vi "Build Rx UDP Engine Configuration.vi"(0 "section ref in":T8=18446744073709551615 format="%.0x", 5 "board properties":T6 {"portConfig" items=["FDX_SINGLE", "FDX_REDUNDANT"]; "portSpeed" items=["FDX_100MBIT", "FDX_10MBIT", "FDX_AUTO_100MBIT", "FDX_AUTO_10MBIT", "FDX_AUTO_ERROR", "FDX_1000MBIT"]}, 9 "port properties":T5, 11 "error in":errorcluster) -> (4 "section ref out":T8 format="%.0x", 6 "boardId":u32, 8 "portId":u32, 10 "VL Configurations":T7(array[cluster]) {"VL Config"."FilterMode" items=["FDX_RX_VL_FLT_DIS", "FDX_RX_VL_FLT_ENA ", "FDX_RX_VL_FLT_ENA_INV"]; "VL Config"."VLBufSize" format="%.0x"; "VL Config"."VerificationMode" items=["FDX_RX_VL_CHECK_ENA_DEFAULT"=65535, "FDX_RX_VL_CHECK_REDMAM"=16, "DX_RX_VL_CHECK_TRAFIC"=8, "FDX_RX_VL_CHECK_FRAMESIZE"=4, "FDX_RX_VL_CHECK_SNINTEG"=2, "FDX_RX_VL_CHECK_INVPAC"=1, "FDX_RX_VL_CHECK_DISA"=0]}, 14 "CommPort Payload":T3[](array[typedef]) {"Parameters"."encoding" items=["BNR", "BCD", "Discrete", "Signed_32", "Signed_64", "Float_32", "Float_64", "Opaque"]}, 15 "error out":errorcluster)   [LabVIEW 2020, in "AIM ARINC 664 Scripting.lvlib"]
uses:
  AIM ARINC 664 Scripting.lvlib
  <vilib>/NI VeriStand/Custom Device API/Custom Device API.lvlib
  Program Files/National Instruments/LabVIEW 2025/instr.lib/AIM GmbH/_AIM 664/_controls/comm_udp_rx.ctl
  Program Files/National Instruments/LabVIEW 2025/instr.lib/AIM GmbH/_AIM 664/AIM664LV.lvlib
  Program Files/National Instruments/LabVIEW 2025/instr.lib/AIM GmbH/_AIM 664/_controls/comm_verification_rx.ctl
  Shared/Encoding (Arinc664).ctl
  Import/_typedefs/frame_parameter_definition.ctl
  Import/AIM ARINC 664 Import.lvlib
  Shared/rx_udp_payload_config.ctl
  <vilib>/NI VeriStand/Custom Device API/Custom Device Item Ref.ctl
  Import/_typedefs/board_setup.ctl
  Import/_typedefs/port_setup.ctl
panel:
  in  "Cluster":cluster{"VL Config":T1, "CommPort Config":T2[]} {"VL Config"."FilterMode" items=["FDX_RX_VL_FLT_DIS", "FDX_RX_VL_FLT_ENA ", "FDX_RX_VL_FLT_ENA_INV"]; "VL Config"."VLBufSize" format="%.0x"; "VL Config"."VerificationMode" items=["FDX_RX_VL_CHECK_ENA_DEFAULT"=65535, "FDX_RX_VL_CHECK_REDMAM"=16, "DX_RX_VL_CHECK_TRAFIC"=8, "FDX_RX_VL_CHECK_FRAMESIZE"=4, "FDX_RX_VL_CHECK_SNINTEG"=2, "FDX_RX_VL_CHECK_INVPAC"=1, "FDX_RX_VL_CHECK_DISA"=0]}
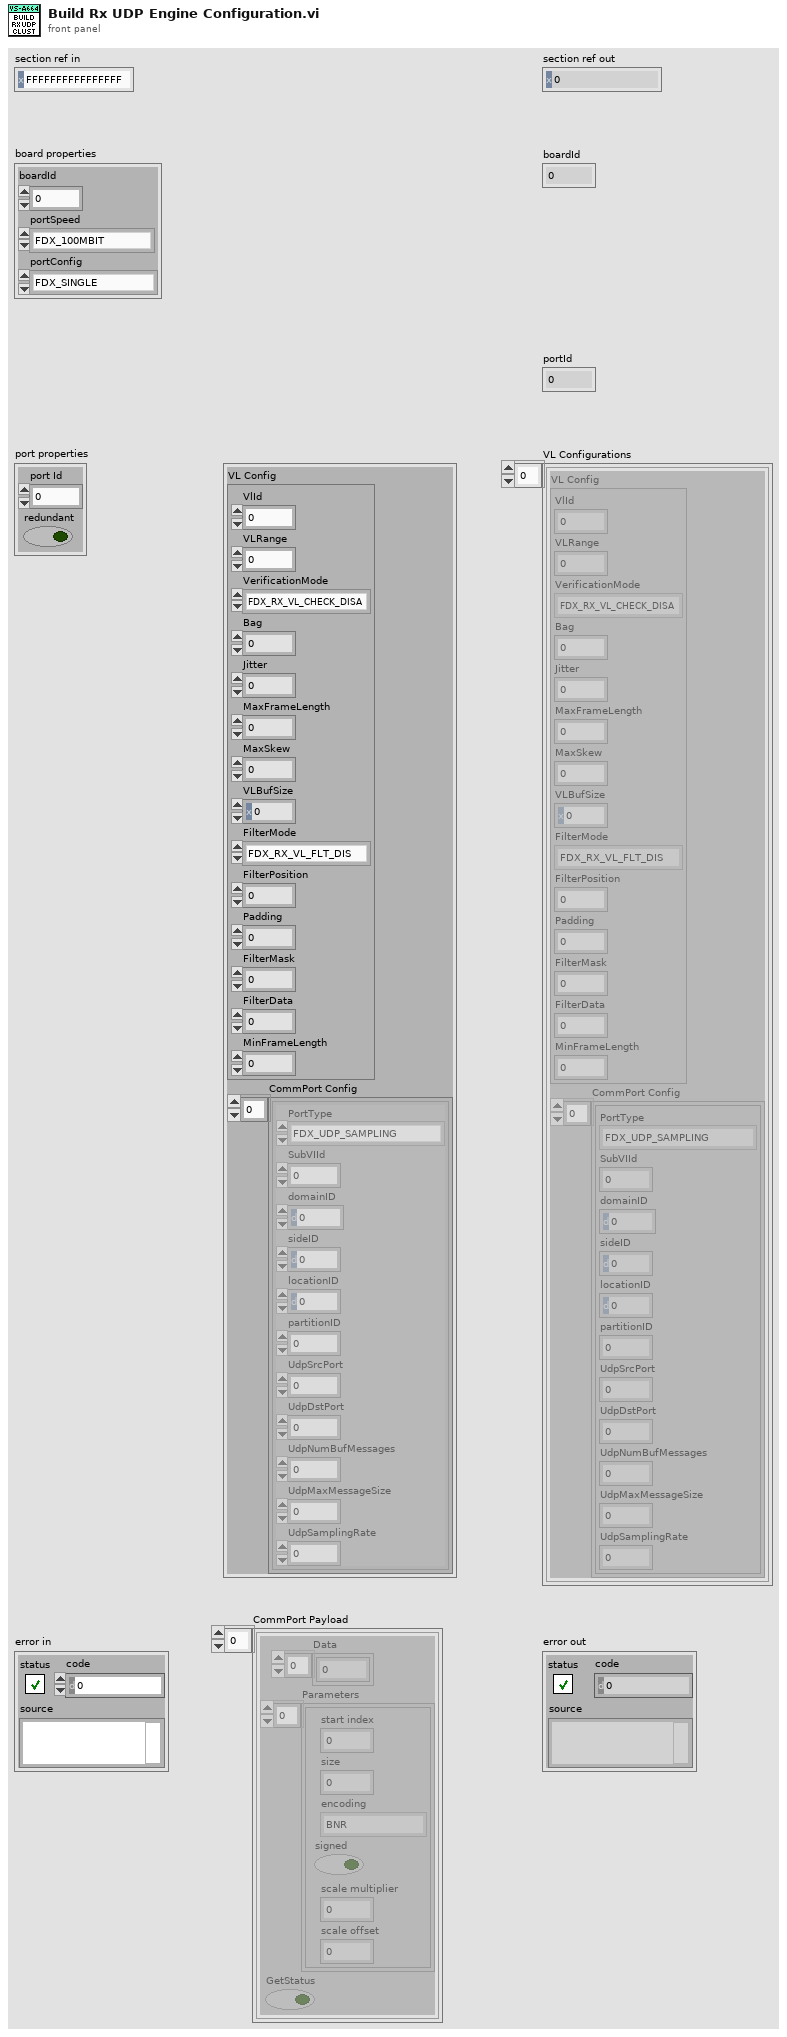
[diagram p1: front panel]
types:
  T1 = typedef "AIM664LV.lvlib/comm_verification_rx.ctl" = cluster{"VlId":u16, "VLRange":u32, "VerificationMode":u32, "Bag":u32, "Jitter":u32, "MaxFrameLength":u32, "MaxSkew":u32, "VLBufSize":u32, "FilterMode":u32, "FilterPosition":u32, "Padding":u32, "FilterMask":u32, "FilterData":u32, "MinFrameLength":u32}
  T2 = typedef "AIM664LV.lvlib/comm_udp_rx.ctl" = cluster{"PortType":enum16{"FDX_UDP_SAMPLING", "FDX_UDP_QUEUING"}, "SubVIId":u32, "domainID":u8, "sideID":u8, "locationID":u8, "partitionID":u8, "UdpSrcPort":u16, "UdpDstPort":u16, "UdpNumBufMessages":u32, "UdpMaxMessageSize":u32, "UdpSamplingRate":u32}
  T3 = typedef "rx_udp_payload_config.ctl" = cluster{"Data":u8[], "Parameters":cluster{"start index":i32, "size":i32, "encoding":T4, "signed":bool, "scale multiplier":dbl, "scale offset":dbl}[], "GetStatus":bool}
  T4 = typedef "Encoding (Arinc664).ctl" = u16
  T5 = typedef "AIM ARINC 664 Import.lvlib/port_setup.ctl" = cluster{"port Id":u32, "redundant":bool}
  T6 = typedef "AIM ARINC 664 Import.lvlib/board_setup.ctl" = cluster{"boardId":u32, "portSpeed":u32, "portConfig":u32}
  T7 = cluster{"VL Config":T1, "CommPort Config":T2[]}[]
  T8 = typedef "Custom Device API.lvlib/Custom Device Item Ref.ctl" = u64
  T9 = typedef "AIM ARINC 664 Import.lvlib/frame_parameter_definition.ctl" = cluster{"start index":i32, "size":i32, "encoding":T4, "signed":bool, "scale multiplier":dbl, "scale offset":dbl}
  T10 = typedef "Custom Device API.lvlib/Custom Device Item Info.ctl" = cluster{"Name":string, "Is Channel":bool, "GUID":string, "Is Waveform":bool}
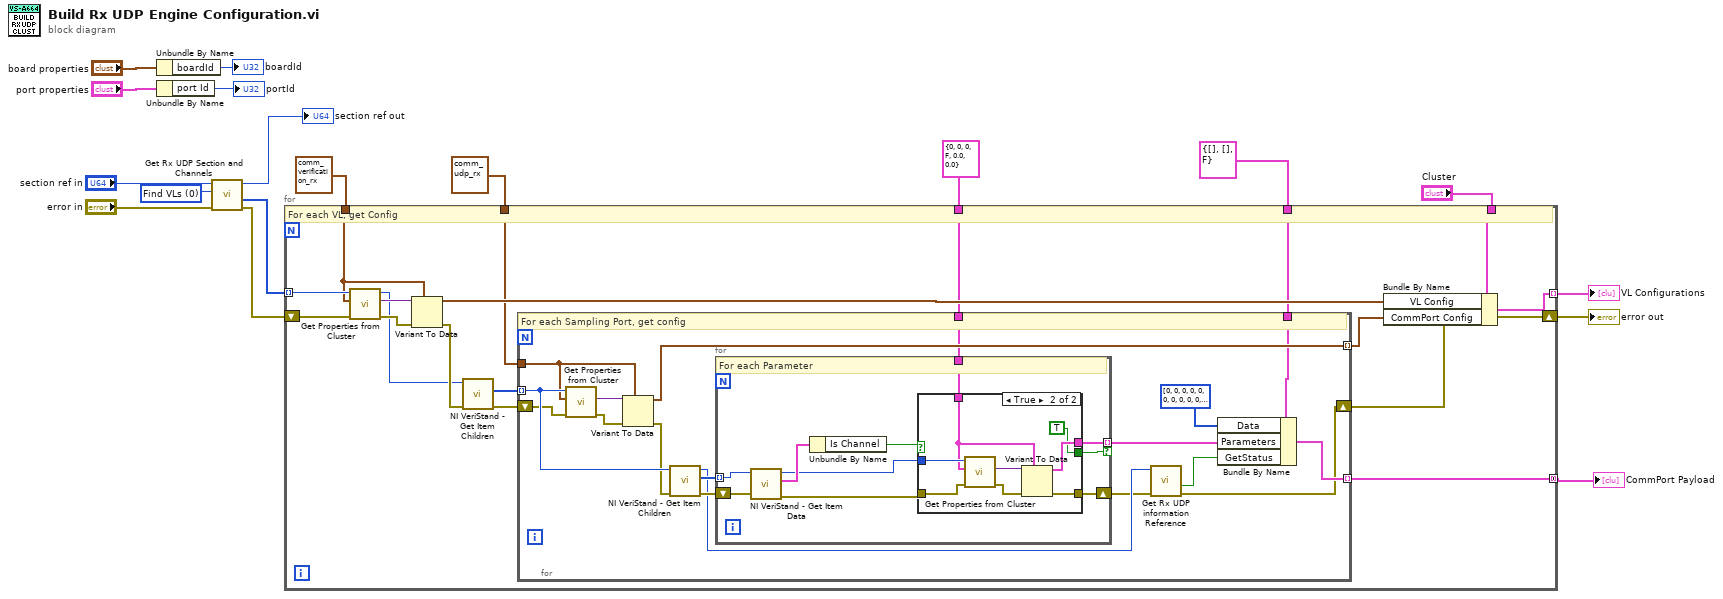
[diagram p0: block diagram]
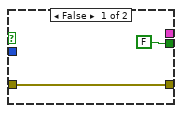
[diagram p2: hidden frame]
diagram:
  w5 = u16 0 items=["Find VLs", "Find Parameters"] ("Option")
  n1 = Unbundle By Name("board properties") -> ("boardId"=→"boardId":u32)
  n2 = Unbundle By Name("port properties") -> ("port Id"=→"portId":u32)
  n3 = call "Get Rx UDP Section and Channels.vi"("error in"="error in", "option"=w5, "custom device ref in"="section ref in") -> ("error out"=w8:errorcluster, "Rx UDP channel refs"=w4:T8[], "custom device ref out"=→"section ref out":T8)  [unwired: 4 in, 2 out]
  n4 = for {
    tunnel: [w28] -> w10 mode=indexing
    shift-right: [w26] -> w11
    shift-left: w8 -> [w36]
    tunnel: [w19] -> w1 mode=concatenating
    tunnel: w4 -> [w25] mode=indexing
    tunnel: "Cluster" -> [w24]
    tunnel: T2 {"PortType"=enum."FDX_UDP_SAMPLING", "SubVIId"=0, "domainID"=1, "sideID"=1, "locationID"=1, "partitionID"=1, "UdpSrcPort"=0, "UdpDstPort"=0, "UdpNumBufMessages"=0, "UdpMaxMessageSize"=0, "UdpSamplingRate"=0} ("CommPort Config") -> [w23]
    tunnel: T1 {"VlId"=0, "VLRange"=0, "VerificationMode"=0, "Bag"=0, "Jitter"=0, "MaxFrameLength"=0, "MaxSkew"=0, "VLBufSize"=32768, "FilterMode"=0, "FilterPosition"=0, "Padding"=0, "FilterMask"=0, "FilterData"=0, "MinFrameLength"=0} ("VL Config") -> [w22]
    tunnel: T9 {"start index"=0, "size"=0, "encoding"=0, "signed"=FALSE, "scale multiplier"=0.0, "scale offset"=0.0} ("Parameter 2") -> [w21]
    tunnel: T3 {"Data"=[], "Parameters"=[], "GetStatus"=FALSE} ("CommPort Payload") -> [w20]
    # "For each VL, get Config"
    n5 = call "Get Properties from Cluster.vi"("error in"=w36, "Variant Cluster"=w22, "custom device ref in"=w25) -> ("error out"=w34:errorcluster, "data"=w35:variant, "custom device ref out"=w32:T8)  [unwired: 5 in, 1 out]
    n6 = Variant To Data(error in=w34, type=w22, Variant=w35) -> (data=w29:T1, error out=w33:errorcluster)
    n7 = call <vilib>:"NI VeriStand - Get Item Children.vi"("error in (no error)"=w33, "Item Ref in"=w32) -> ("error out"=w30:errorcluster, "Child Refs"=w31:T8[])  [unwired: 6 in, 2 out]
    n8 = for {
      tunnel: w31 -> [w50] mode=indexing
      shift-right: [w37] -> w26
      shift-left: w30 -> [w46]
      tunnel: [w49] -> w27 mode=indexing
      tunnel: [w47] -> w19 mode=indexing
      tunnel: w23 -> [w44]
      tunnel: w21 -> [w43]
      tunnel: w20 -> [w42]
      # "For each Sampling Port, get config"
      n9 = call "Get Properties from Cluster.vi"("error in"=w46, "Variant Cluster"=w44, "custom device ref in"=w50) -> ("error out"=w52:errorcluster, "data"=w51:variant)  [unwired: 5 in, 2 out]
      n10 = Variant To Data(error in=w52, type=w44, Variant=w51) -> (data=w49:T2, error out=w45:errorcluster)
      n11 = call <vilib>:"NI VeriStand - Get Item Children.vi"("error in (no error)"=w45, "Item Ref in"=w50) -> ("error out"=w53:errorcluster, "Child Refs"=w54:T8[], "Item Ref out"=w39:T8)  [unwired: 6 in, 1 out]
      n12 = for {
        tunnel: w54 -> [w59] mode=indexing
        shift-right: [w63] -> w38
        shift-left: w53 -> [w60]
        tunnel: [w64] -> w48 mode=indexing if=w55
        tunnel: w43 -> [w62]
        # "For each Parameter"
        n13 = call <vilib>:"NI VeriStand - Get Item Data.vi"("error in (no error)"=w60, "Item Ref in"=w59) -> ("error out"=w58:errorcluster, "Item Info"=w61:T10, "Item Ref out"=w57:T8)  [unwired: 7 out]
        n14 = Unbundle By Name(w61) -> ("Is Channel"=w56:bool)
        n15 = case shown="True" w56 {
          tunnel: w57 -> [_ w72]
          tunnel: [_ w71] -> w64
          tunnel: w58 -> [w65 w70]
          tunnel: [w65 w69] -> w63
          tunnel: w62 -> [_ w68]
          tunnel: [FALSE TRUE] -> w55
          frame False {
          }
          frame True {
            n16 = call "Get Properties from Cluster.vi"("error in"=w70, "Variant Cluster"=w68, "custom device ref in"=w72) -> ("error out"=w73:errorcluster, "data"=w74:variant)  [unwired: 5 in, 2 out]
            n17 = Variant To Data(error in=w73, type=w68, Variant=w74) -> (data=w71:T9, error out=w69:errorcluster)
          }
        }
      }
      n18 = call "Get Rx UDP information Reference.vi"("error in"=w38, "custom device ref"=w39) -> ("error out"=w37:errorcluster, "found?"=w40:bool)  [unwired: 7 in, 1 out]
      n19 = Bundle By Name(cluster=w42, "Data"=u8[] [0, 0, 0, 0, 0, 0, 0, 0, 0, 0, 0, 0, 0, 0, 0, 0, 0, 0, 0, 0, 0, 0, 0, 0, 0, 0, 0, 0, 0, 0, 0, 0, 0, 0, 0, 0, 0, 0, 0, 0, 0, 0, 0, 0, 0, 0, 0, 0, 0, 0, 0, 0, 0, 0, 0, 0, 0, 0, 0, 0, 0, 0, 0, 0, 0, 0, 0, 0, 0, 0, 0, 0, 0, 0, 0, 0, 0, 0, 0, 0, 0, 0, 0, 0, 0, 0, 0, 0, 0, 0, 0, 0, 0, 0, 0, 0, 0, 0, 0, 0, 0, 0, 0, 0, 0, 0, 0, 0, 0, 0, 0, 0, 0, 0, 0, 0, 0, 0, 0, 0, 0, 0, 0, 0, 0, 0, 0, 0, 0, 0, 0, 0, 0, 0, 0, 0, 0, 0, 0, 0, 0, 0, 0, 0, 0, 0, 0, 0, 0, 0, 0, 0, 0, 0, 0, 0, 0, 0, 0, 0, 0, 0, 0, 0, 0, 0, 0, 0, 0, 0, 0, 0, 0, 0, 0, 0, 0, 0, 0, 0, 0, 0, 0, 0, 0, 0, 0, 0, 0, 0, 0, 0, 0, 0, 0, 0, 0, 0, 0, 0, 0, 0, 0, 0, 0, 0, 0, 0, 0, 0, 0, 0, 0, 0, 0, 0, 0, 0, 0, 0, 0, 0, 0, 0, 0, 0, 0, 0, 0, 0, 0, 0, 0, 0, 0, 0, 0, 0, 0, 0, 0, 0, 0, 0, 0, 0, 0, 0, 0, 0, 0, 0, 0, 0, 0, 0, 0, 0, 0, 0, 0, 0, 0, 0, 0, 0, 0, 0, 0, 0, 0, 0, 0, 0, 0, 0, 0, 0, 0, 0, 0, 0, 0, 0, 0, 0, 0, 0, 0, 0, 0, 0, 0, 0, 0, 0, 0, 0, 0, 0, 0, 0, 0, 0, 0, 0, 0, 0, 0, 0, 0, 0, 0, 0, 0, 0, 0, 0, 0, 0, 0, 0, 0, 0, 0, 0, 0, 0, 0, 0, 0, 0, 0, 0, 0, 0, 0, 0, 0, 0, 0, 0, 0, 0, 0, 0, 0, 0, 0, 0, 0, 0, 0, 0, 0, 0, 0, 0, 0, 0, 0, 0, 0, 0, 0, 0, 0, 0, 0, 0, 0, 0, 0, 0, 0, 0, 0, 0, 0, 0, 0, 0, 0, 0, 0, 0, 0, 0, 0, 0, 0, 0, 0, 0, 0, 0, 0, 0, 0, 0, 0, 0, 0, 0, 0, 0, 0, 0, 0, 0, 0, 0, 0, 0, 0, 0, 0, 0, 0, 0, 0, 0, 0, 0, 0, 0, 0, 0, 0, 0, 0, 0, 0, 0, 0, 0, 0, 0, 0, 0, 0, 0, 0, 0, 0, 0, 0, 0, 0, 0, 0, 0, 0, 0, 0, 0, 0, 0, 0, 0, 0, 0, 0, 0, 0, 0, 0, 0, 0, 0, 0, 0, 0, 0, 0, 0, 0, 0, 0, 0, 0, 0, 0, 0, 0, 0, 0, 0, 0, 0, 0, 0, 0, 0, 0, 0, 0, 0, 0, 0, 0, 0, 0, 0, 0, 0, 0, 0, 0, 0, 0, 0, 0, 0, 0, 0, 0, 0, 0, 0, 0, 0, 0, 0, 0, 0, 0, 0, 0, 0, 0, 0, 0, 0, 0, 0, 0, 0, 0, 0, 0, 0, 0, 0, 0, 0, 0, 0, 0, 0, 0, 0, 0, 0, 0, 0, 0, 0, 0, 0, 0, 0, 0, 0, 0, 0, 0, 0, 0, 0, 0, 0, 0, 0, 0, 0, 0, 0, 0, 0, 0, 0, 0, 0, 0, 0, 0, 0, 0, 0, 0, 0, 0, 0, 0, 0, 0, 0, 0, 0, 0, 0, 0, 0, 0, 0, 0, 0, 0, 0, 0, 0, 0, 0, 0, 0, 0, 0, 0, 0, 0, 0, 0, 0, 0, 0, 0, 0, 0, 0, 0, 0, 0, 0, 0, 0, 0, 0, 0, 0, 0, 0, 0, 0, 0, 0, 0, 0, 0, 0, 0, 0, 0, 0, 0, 0, 0, 0, 0, 0, 0, 0, 0, 0, 0, 0, 0, 0, 0, 0, 0, 0, 0, 0, 0, 0, 0, 0, 0, 0, 0, 0, 0, 0, 0, 0, 0, 0, 0, 0, 0, 0, 0, 0, 0, 0, 0, 0, 0, 0, 0, 0, 0, 0, 0, 0, 0, 0, 0, 0, 0, 0, 0, 0, 0, 0, 0, 0, 0, 0, 0, 0, 0, 0, 0, 0, 0, 0, 0, 0, 0, 0, 0, 0, 0, 0, 0, 0, 0, 0, 0, 0, 0, 0, 0, 0, 0, 0, 0, 0, 0, 0, 0, 0, 0, 0, 0, 0, 0, 0, 0, 0, 0, 0, 0, 0, 0, 0, 0, 0, 0, 0, 0, 0, 0, 0, 0, 0, 0, 0, 0, 0, 0, 0, 0, 0, 0, 0, 0, 0, 0, 0, 0, 0, 0, 0, 0, 0, 0, 0, 0, 0, 0, 0, 0, 0, 0, 0, 0, 0, 0, 0, 0, 0, 0, 0, 0, 0, 0, 0, 0, 0, 0, 0, 0, 0, 0, 0, 0, 0, 0, 0, 0, 0, 0, 0, 0, 0, 0, 0, 0, 0, 0, 0, 0, 0, 0, 0, 0, 0, 0, 0, 0, 0, 0, 0, 0, 0, 0, 0, 0, 0, 0, 0, 0, 0, 0, 0, 0, 0, 0, 0, 0, 0, 0, 0, 0, 0, 0, 0, 0, 0, 0, 0, 0, 0, 0, 0, 0, 0, 0, 0, 0, 0, 0, 0, 0, 0, 0, 0, 0, 0, 0, 0, 0, 0, 0, 0, 0, 0, 0, 0, 0, 0, 0, 0, 0, 0, 0, 0, 0, 0, 0, 0, 0, 0, 0, 0, 0, 0, 0, 0, 0, 0, 0, 0, 0, 0, 0, 0, 0, 0, 0, 0, 0, 0, 0, 0, 0, 0, 0, 0, 0, 0, 0, 0, 0, 0, 0, 0, 0, 0, 0, 0, 0, 0, 0, 0, 0, 0, 0, 0, 0, 0, 0, 0, 0, 0, 0, 0, 0, 0, 0, 0, 0, 0, 0, 0, 0, 0, 0, 0, 0, 0, 0, 0, 0, 0, 0, 0], "Parameters"=w48, "GetStatus"=w40) -> (w47:T3)
    }
    n20 = Bundle By Name(cluster=w24, "VL Config"=w29, "CommPort Config"=w27) -> (w28:cluster{"VL Config":T1, "CommPort Config":T2[]})
  }
  "error out" <- w11
  "VL Configurations" <- w10
  "CommPort Payload" <- w1
